vi "CloseFile.vi"(8 "error in (no error)":errorcluster, 11 "FileMerge in":refnum<class "FileMerge.lvclass">) -> (0 "error out":errorcluster, 3 "FileMerge out":refnum<class "FileMerge.lvclass">)   [LabVIEW 2019, in "FileMerge.lvclass"]
doc: "Finish up merged file.\nIf there's data at the end of the original file, and we're done with the new data acqisition and merging, copy over the rest of the original file.\nMake sure the merged file has the ENDOFFILE keyword at the end."
uses:
  FileMerge.lvclass
  FileMerge.lvclass/FileMerge.ctl
  ExistingFileMgr/ExistingFileMgr.lvclass
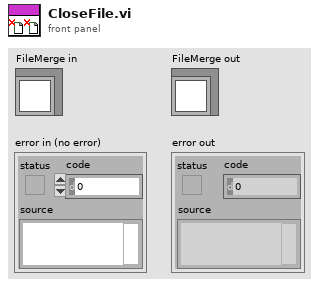
[diagram p1: front panel]
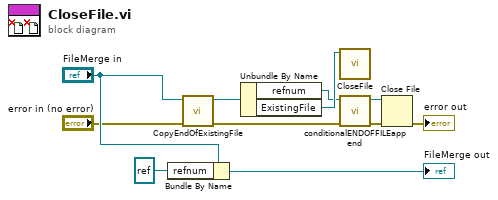
[diagram p0: block diagram]
diagram:
  n1 = Bundle By Name(cluster="FileMerge in", "refnum"=refnum<file> refnum) -> (→"FileMerge out":refnum<class "FileMerge.lvclass">)
  n2 = call "CopyEndOfExistingFile.vi"("error in (no error)"="error in (no error)", "FileMerge in"="FileMerge in") -> ("error out"=w1:errorcluster, "FileMerge out"=w7:refnum<class "FileMerge.lvclass">)  [unwired: 8 in]
  n3 = Unbundle By Name(w7) -> ("refnum"=w4:refnum<file>, "ExistingFile"=w10:refnum<class "ExistingFileMgr.lvclass">)
  n4 = call "CloseFile.vi"("ExistingFileMgr in"=w10) -> ()  [unwired: 9 in, 2 out]
  n5 = call "conditionalENDOFFILEappend.vi"("error in"=w1, "refnum"=w4) -> ("error out"=w2:errorcluster, "refnum out"=w3:refnum<file>)  [unwired: 8 in]
  n6 = Close File(refnum=w3, error in=w2) -> (error out=→"error out":errorcluster)  [unwired: 1 out]
